vi "impulse_filter_distance.vi"(11 "Delta":sgl[](array[numeric])) -> (3 "Distance":sgl)   [LabVIEW 2013]
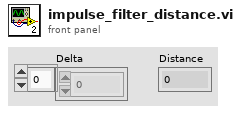
[diagram p1: front panel]
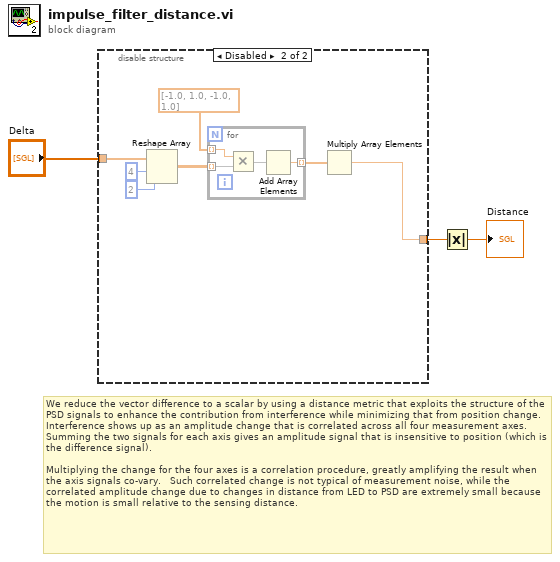
[diagram p0: block diagram]
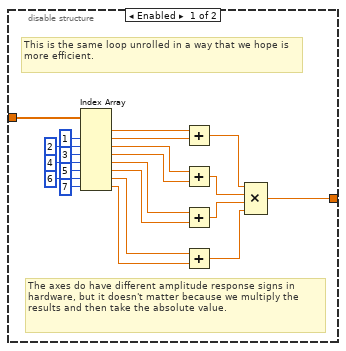
[diagram p2: hidden frame]
diagram:
  # "We reduce the vector difference to a scalar by using a distance metric that exploits the structure of the PSD signals to enhance the contribution from interference while minimizing that from position change.    Interference shows up as an amplitude change that is correlated across all four measurement axes.   Summing the two signals for each axis gives an amplitude signal that is insensitive to position (which is the difference signal).    \n\nMultiplying the change for the four axes is a correlation procedure, greatly amplifying the result when the axis signals co-vary.   Such correlated change is not typical of measurement noise, while the correlated amplitude change due to changes in distance from LED to PSD are extremely small because the motion is small relative to the sensing distance."
  n1 = disable-structure shown="Disabled" {
    disable-tunnel: [w6 w31] -> w1
    disable-tunnel: "Delta" -> [w17 w26]
    frame Enabled {
      # "The axes do have different amplitude response signs in hardware, but it doesn't matter because we multiply the results and then take the absolute value."
      # "This is the same loop unrolled in a way that we hope is more efficient."
      n2 = Index Array(array=w17, index #2=1 ("index"), index #3=2 ("index"), index #4=3 ("index"), index #5=4 ("index"), index #6=5 ("index"), index #7=6 ("index"), index #8=7 ("index")) -> (element #1=w10:sgl, element #2=w9:sgl, element #3=w16:sgl, element #4=w15:sgl, element #5=w8:sgl, element #6=w7:sgl, element #7=w14:sgl, element #8=w13:sgl)  [unwired: 1 in]
      n3 = Add(x=w10, y=w9) -> (x+y=w4:sgl)
      n4 = Add(x=w16, y=w15) -> (x+y=w12:sgl)
      n5 = Add(x=w8, y=w7) -> (x+y=w5:sgl)
      n6 = Add(x=w14, y=w13) -> (x+y=w11:sgl)
      n7 = Compound Arithmetic op=MULTIPLY(w4, w12, w5, w11) -> (w6:sgl)
    }
    frame Disabled {
      n8 = Reshape Array(w26, 4 ("dimension size"), 2 ("dimension size")) -> (w29:sgl[][])
      n9 = for {
        tunnel: sgl[] [-1.0, 1.0, -1.0, 1.0] ("x-y") -> [w35] mode=indexing
        tunnel: w29 -> [w34] mode=indexing
        tunnel: [w32] -> w30 mode=indexing
        n10 = Multiply(x=w35, y=w34) -> (x*y=w33:sgl[])
        n11 = Add Array Elements(numeric array=w33) -> (sum=w32:sgl)
      }
      n12 = Multiply Array Elements(1:w30) -> (0:w31:sgl)
    }
  }
  n13 = Absolute Value(x=w1) -> (abs(x)=→"Distance":sgl)
